vi "MainFPGA_APA.vi"() -> ()   [LabVIEW 2019]
uses:
  <vilib>/rvi/Emulation/niFpgaGetClockAttributes.vi
  <vilib>/rvi/Emulation/niFpgaSctlEmulationGetInTimedLoop.vi
  <vilib>/rvi/Emulation/niFpgaEmulationReportErrorSimple.vi
  <vilib>/rvi/eio/common/nirviEmuTemplateMethod_errors.vi
  <vilib>/rvi/Emulation/niFpgaCriticalErrorInLSC.vi
  <vilib>/eio/EIONode/EIONode.xnode
panel:
  in  "A_Digit3":bool
  in  "stop":bool
  in  "A_Digit0":bool
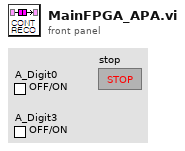
[diagram p1: front panel]
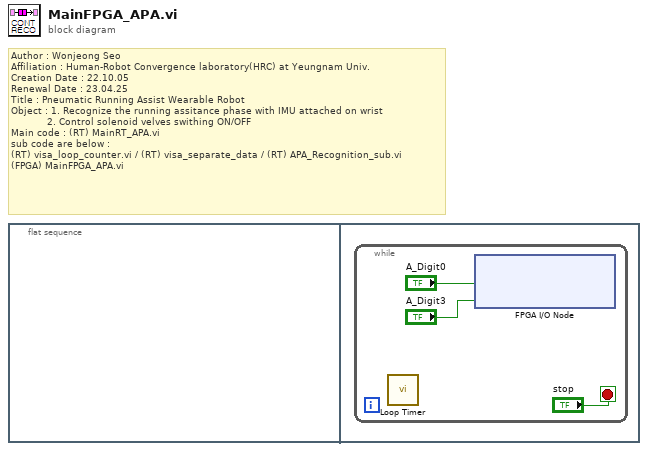
[diagram p0: block diagram]
diagram:
  # "Author : Wonjeong Seo\nAffiliation : Human-Robot Convergence laboratory(HRC) at Yeungnam Univ.\nCreation Date : 22.10.05\nRenewal Date : 23.04.25\nTitle : Pneumatic Running Assist Wearable Robot\nObject : 1. Recognize the running assitance phase with IMU attached on wrist\n            2. Control solenoid velves swithing ON/OFF\nMain code : (RT) MainRT_APA.vi\nsub code are below :\n(RT) visa_loop_counter.vi / (RT) visa_separate_data / (RT) APA_Recognition_sub.vi\n(FPGA) MainFPGA_APA.vi"
  n1 = flat-sequence {
    frame #0 {
    }
    frame #1 {
      n2 = while {
        stop <- "stop" stop-if-true
        n3 = call "Loop Timer"() -> ()  [unwired: 1 in, 1 out]
        n4 = xnode "FPGA I/O Node"("ConnectorA/DIO0"="A_Digit0", "ConnectorA/DIO3"="A_Digit3") -> ()  [unwired: 2 in, 2 out]
      }
    }
  }
